vi "Min Read Single.vi"(8 "error in":errorcluster, 9 "Channel Index":i32=1, 11 "Min Limit in":refnum<class "Limit.lvclass">) -> (0 "error out":errorcluster, 1 "Changed or First Call?":bool, 2 "Current Min SP":dbl, 3 "Min Limit out":refnum<class "Limit.lvclass">)   [LabVIEW 2023, in "Limit.lvclass"]
uses:
  Limit.lvclass
  <vilib>/ADAS Replay HIL/Channels/Tag Wrapper/Tag Wrapper.lvlib
  <vilib>/ADAS Replay HIL/Channels/Tag Wrapper/Polymorphic/Read Channel (Double).vi
  454d93e5-0a74-4a7e-902d-56120c423366.vi
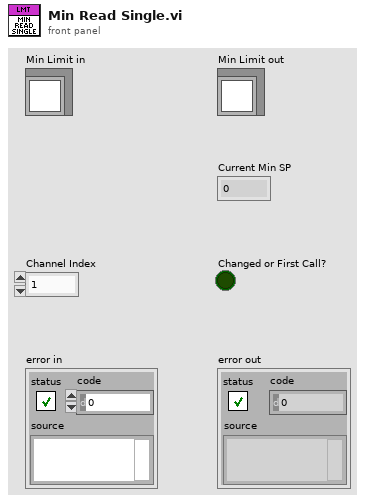
[diagram p1: front panel]
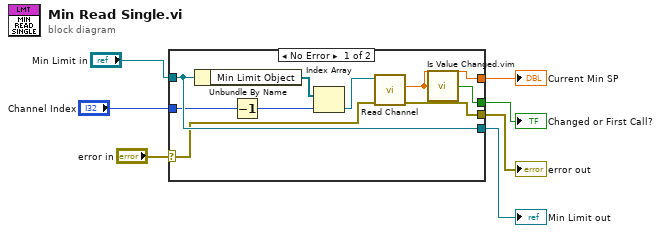
[diagram p0: block diagram]
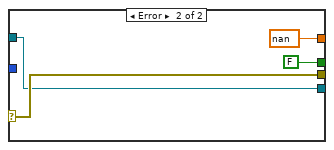
[diagram p2: hidden frame]
diagram:
  n1 = case shown="No Error" "error in" {
    selector: "error in" -> [w14 w20]
    tunnel: [w13 w20] -> w3
    tunnel: [w16 w19] -> w2
    tunnel: "Min Limit in" -> [w16 w19]
    tunnel: [w12 nan] -> w4
    tunnel: [w11 FALSE ("changed or first call?")] -> w1
    tunnel: "Channel Index" -> [w9 _]
    frame No Error {
      n2 = Unbundle By Name(w16) -> ("Min Limit Object"=w15:refnum<k21>[])
      n3 = Decrement(x=w9) -> (x-1=w8:i32)
      n4 = Index Array(array=w15, index=w8) -> (element=w10:refnum<k21>)
      n5 = call-poly <vilib>:"Read Channel.vi"("error in"=w14, "ADAS HIL Channel in"=w10) -> ("error out"=w13:errorcluster, "Value out"=w12:dbl)  [unwired: 6 in, 2 out]
      n6 = call "Is Value Changed.vim"("value"=w12) -> ("changed or first call?"=w11:bool)
    }
    frame Error {
    }
  }
  "error out" <- w3
  "Changed or First Call?" <- w1
  "Current Min SP" <- w4
  "Min Limit out" <- w2
